vi "SharedPlayerCompleted.vi"(1 "Write?":bool, 2 "PlayerCompletedInput":bool) -> (0 "PlayerCompleted":bool)   [LabVIEW 2010, in "Player.lvlib"]
uses:
  Player.lvlib
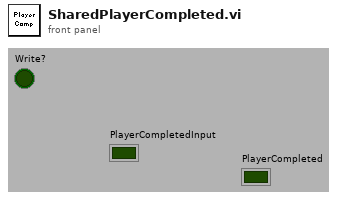
[diagram p1: front panel]
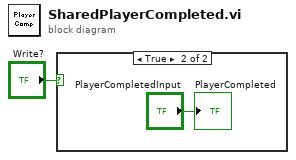
[diagram p0: block diagram]
diagram:
  n1 = case shown="True" "Write?" {
    frame False {
    }
    frame True {
      "PlayerCompleted" <- "PlayerCompletedInput"
    }
  }
